vi "Array2Image.vi"(8 "error in (no error)":errorcluster, 9 "Image Type":T2 items=["Grayscale (U8)", "Grayscale (I16)", "Grayscale (SGL)", "Complex (CSG)", "RGB (U32)", "HSL (U32)", "RGB (U64)", "Grayscale (U16)"], 10 "Image Pixels (U32)":u32[][](array[numeric]), 11 "Image 2":T1) -> (0 "error out":errorcluster, 3 "Image":T1)   [LabVIEW 2017, in "ImageAcquisitionLibrary.lvlib"]
uses:
  ImageAcquisitionLibrary.lvlib
  <vilib>/vision/Image Controls.llb/IMAQ Image.ctl
panel:
  out "Image 3":T1(plugin-control)
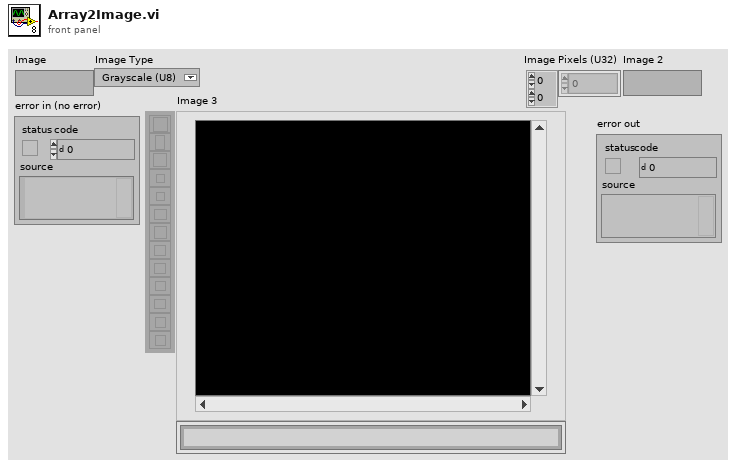
[diagram p1: front panel]
types:
  T1 = typedef "IMAQ Image.ctl" = refnum<image>
  T2 = typedef "Image Type" = u32
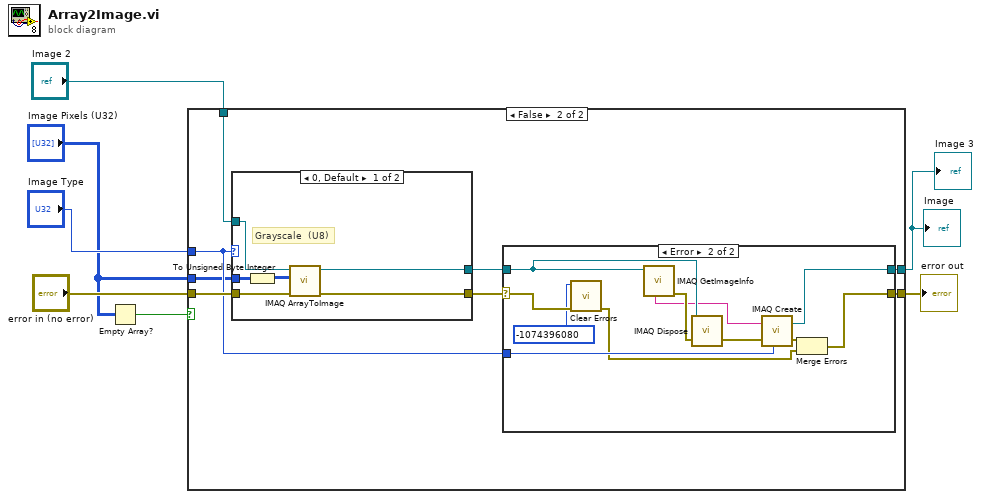
[diagram p0: block diagram]
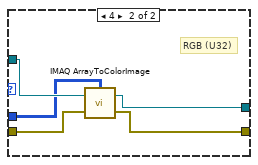
[diagram p4: hidden frame]
diagram:
  n1 = Empty Array?(array="Image Pixels (U32)") -> (empty?=w2:bool)
  n2 = case shown="False" w2 {
    tunnel: "error in (no error)" -> [w8 w17]
    tunnel: "Image 2" -> [w9 w16]
    tunnel: "Image Type" -> [_ w13]
    tunnel: [w9 w12] -> w1
    tunnel: [w8 w11] -> w4
    tunnel: "Image Pixels (U32)" -> [_ w10]
    frame True {
    }
    frame False {
      n3 = case shown="0, Default" w13 {
        tunnel: w17 -> [w36 w39]
        tunnel: [w35 w38] -> w15
        tunnel: w10 -> [w33 w40]
        tunnel: w16 -> [w32 w41]
        tunnel: [w31 w37] -> w14
        frame 0, Default {
          # "Grayscale  (U8)"
          n4 = To Unsigned Byte Integer(number=w33) -> (unsigned 8bit integer=w34:u8[][])
          n5 = call "IMAQ ArrayToImage"("error in (no error)"=w36, "Image Pixels (U8)"=w34, "Image"=w32) -> ("error out"=w35:errorcluster, "Image Out"=w31:T1)  [unwired: 7 in]
        }
        frame 4 {
          # "RGB (U32)"
          n6 = call "IMAQ ArrayToColorImage"("Image Pixels (U32)"=w40, "Image"=w41, "error in (no error)"=w39) -> ("Image Out"=w37:T1, "error out"=w38:errorcluster)  [unwired: 2 in]
        }
      }
      n7 = case shown="Error" w15 {
        selector: w15 -> [w18 w24]
        tunnel: w14 -> [w19 w30]
        tunnel: w13 -> [_ w26]
        tunnel: [w19 w25] -> w12
        tunnel: [w18 w21] -> w11
        frame No Error {
        }
        frame Error {
          n8 = call <vilib>:"Clear Errors.vi"("error in (no error)"=w24, "specific error code to clear (0: all)"=-1074396080) -> ("error out"=w20:errorcluster)  [unwired: 4 in, 1 out]
          n9 = call "IMAQ GetImageInfo"("Image"=w30) -> ("error out"=w29:errorcluster, "Image Name"=w27:string)  [unwired: 3 in, 6 out]
          n10 = call "IMAQ Dispose"("Image"=w30, "error in (no error)"=w29) -> ("error out"=w28:errorcluster)  [unwired: 4 in]
          n11 = call "IMAQ Create"("Image Name"=w27, "Image Type"=w26, "error in (no error)"=w28) -> ("New Image"=w25:T1, "error out"=w22:errorcluster)  [unwired: 2 in]
          n12 = Merge Errors(w22, w20) -> (w21:errorcluster)
        }
      }
    }
  }
  "Image" <- w1
  "error out" <- w4
  "Image 3" <- w1
